vi "Read Notifier User Event.vi"(8 "error in (no error)":errorcluster, 11 "QTab Class in":refnum<class "QTab Class.lvclass">) -> (0 "error out":errorcluster, 2 "Notifier User Event":T1, 3 "QTab Class out":refnum<class "QTab Class.lvclass">)   [LabVIEW 2020, in "QTab.lvlib" / "QTab Class.lvclass"]
uses:
  QTab Class.lvclass
  Notifier User Event.ctl
  QTab Class.lvclass/QTab Class.ctl
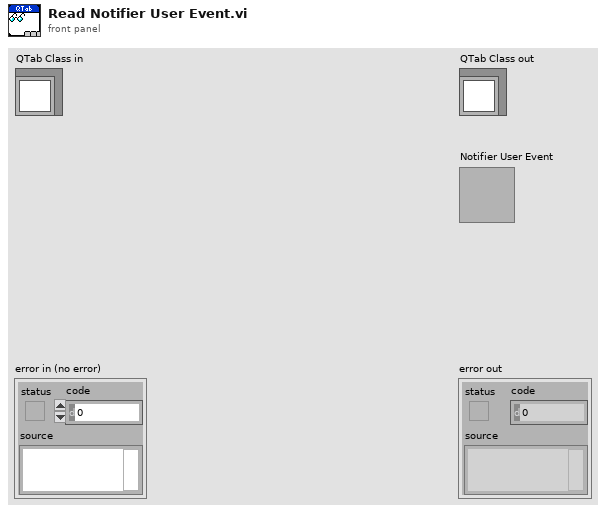
[diagram p1: front panel]
types:
  T1 = typedef "QTab.lvlib/QTab Class.lvclass/Notifier User Event.ctl" = cluster{"Close User Event":refnum<user-event>}
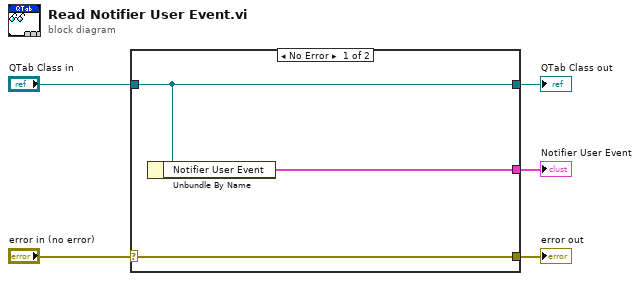
[diagram p0: block diagram]
diagram:
  n1 = case shown="No Error" "error in (no error)" {
    selector: "error in (no error)" -> [w8 w9]
    tunnel: [w8 w9] -> w4
    tunnel: [w7 w10] -> w2
    tunnel: "QTab Class in" -> [w7 w10]
    tunnel: [w6 _] -> w1
    frame No Error {
      n2 = Unbundle By Name(w7) -> ("Notifier User Event"=w6:T1)
    }
    frame Error {
    }
  }
  "error out" <- w4
  "QTab Class out" <- w2
  "Notifier User Event" <- w1
